vi "SubModule Config.vi"(6 "Status":bool, 8 "error in (no error)":errorcluster, 9 "Cycles":i32, 10 "Name":string, 11 "Canon in":refnum<class "Canon.lvclass">) -> (0 "error out":errorcluster, 3 "Canon out":refnum<class "Canon.lvclass">)   [LabVIEW 2021, in "Canon.lvclass"]
uses:
  Canon.lvclass
  C:/Projects/InstrPanel/Classes/Camera/Camera.lvclass
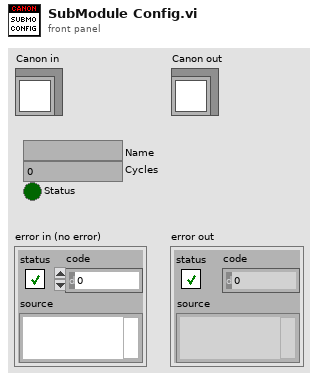
[diagram p1: front panel]
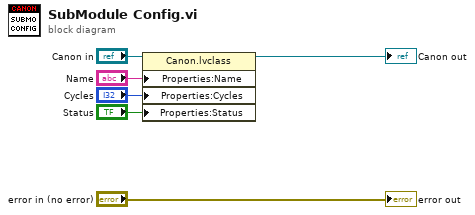
[diagram p0: block diagram]
diagram:
  n1 = property class="Canon.lvclass"(reference="Canon in", "Properties:Name"="Name", "Properties:Cycles"="Cycles", "Properties:Status"="Status") -> (reference out=→"Canon out":refnum<class "Canon.lvclass">)  [unwired: 1 in, 1 out]
  "error out" <- "error in (no error)"
